vi "Day 6.vi"() -> ()   [LabVIEW 2023]
uses:
  666ad4e4-d0b9-4e2d-b008-2c230202d64d.vi
panel:
  in  "Marker length":i32=4
  out "Answer":i32
  out "Marker":string
  in  "input":string="lrdrgrcggjrgrddfqfqrqppptrtssnqqqlzqqslspppsddfnnwgnnwhhjttnsnswnnbqbrrcqrqdqcdddlnddwwlmmlmtmwmggjgjmmmrppqhhswhwhmhchtchhsttvbtvvpspjjqrrgqrqmqvmvzmvzzrnnqlnlwlttjstjtjvjddrzzrnrmrbmbwwzppnqpqmmjnnvqnvvdzdpdvvmhvhhmshmsssvnnqppclcqlcqctqtfffvrfvrffptfftppncncwnntfntftdftfhfzzfwzzcddngdndccrttjmmcddrvrwwnntggghccjbjvbvjvlvjlvlgljlnjjtvjjfddmwwhnnqnrnccwllpmprmmspsvsrsslstsllpmllfzlflqltlssdbbdsdqsdqqgfgfjjtzjzmmsnsmnnzssgfgzgjgwwqfqtfthhhczzpwprwwqttqcqctcpcrrvwrvrggfvfqvvbqqhnnczcjjjfbfhbhjhssnwwfswszwwgbgzgczcbbvmvrrdgrddfwdffvsvtstztftfvfssgffnrnnzzqddltdtbdttnnfrnnfrfddpmpqqplqqbdbzbnnnrt..."
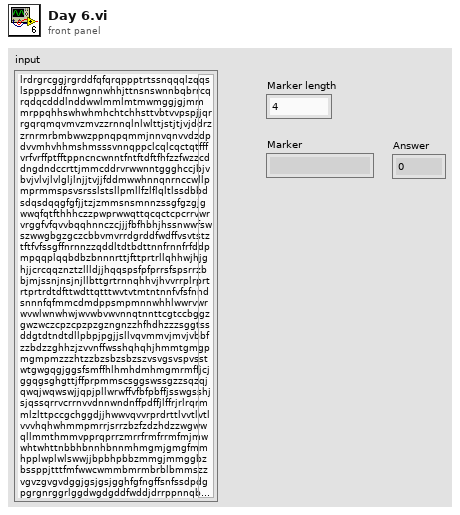
[diagram p1: front panel]
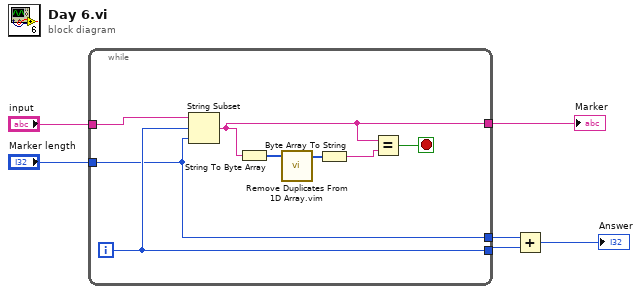
[diagram p0: block diagram]
diagram:
  n1 = while {
    tunnel: "input" -> [w14]
    tunnel: [w11] -> w3
    tunnel: [w8] -> w5
    tunnel: "Marker length" -> [w7]
    tunnel: [w7] -> w1
    i -> [w8]
    stop <- w9 stop-if-true
    n2 = String Subset(string=w14, offset (0)=w8, length (rest)=w7) -> (substring=w11:string)
    n3 = String To Byte Array(string=w11) -> (unsigned byte array=w13:u8[])
    n4 = call "Remove Duplicates From 1D Array.vim"("array"=w13) -> ("array with duplicates removed"=w12:u8[])  [unwired: 10 in]
    n5 = Byte Array To String(unsigned byte array=w12) -> (string=w10:string)
    n6 = Equal?(x=w11, y=w10) -> (x = y?=w9:bool)
  }
  "Marker" <- w3
  n7 = Add(x=w1, y=w5) -> (x+y=→"Answer":i32)
